vi "Cannon Set.vi"(1 "Cannon Global Data In":T1) -> (0 "Cannon Global Data Out":T1)   [LabVIEW 2012]
uses:
  <vilib>/Rock Robotics/WPI/DriverStation/WPI_DriverStationRobotMode2.ctl
  Extras/Global Data.vi
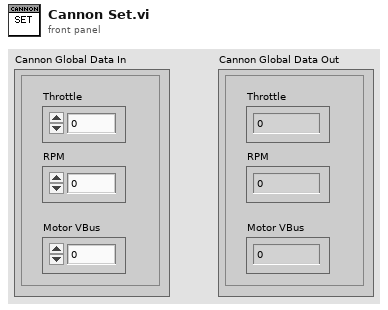
[diagram p1: front panel]
types:
  T1 = cluster{"Throttle":dbl, "RPM":dbl, "Motor VBus":dbl}
  T2 = typedef "WPI_DriverStationRobotMode2.ctl" = enum16{"Autonomous Disabled", "Autonomous Enabled", "Teleop Disabled", "Teleop Enabled", "Timeout", "Finish", "Test Disabled", "Test Enabled"}
  T3 = typedef "WPI_MotorControlDeviceRef.ctl" = cluster{"DeviceStatus":errorcluster, "Type":enum16{"PWM", "CAN"}, "PWM":cluster{"Digital Module":T4, "PWM Channel":T5, "DeadBand":T6}, "CAN":cluster{"Device Number":u8, "Control Mode":T7, "Semaphore":T8, "Max Vout":dbl}, "Invert":bool, "TransformRef":T9, "InvTransformRef":T9}
  T4 = typedef "FPGA_TypedefDigitalModule.ctl" = enum16{"Digital Module 1", "Digital Module 2"}
  T5 = typedef "FPGA_DIOPWMChannel.ctl" = enum8{"PWM 1", "PWM 2", "PWM 3", "PWM 4", "PWM 5", "PWM 6", "PWM 7", "PWM 8", "PWM 9", "PWM 10", "Invalid"}
  T6 = typedef "WPI_PWMDeadband.ctl" = cluster{"Name":string, "maxPositivePwm":i32, "minPositivePwm":i32, "centerPwm":i32, "maxNegativePwm":i32, "minNegativePwm":i32, "angularRange":u16}
  T7 = typedef "WPI_CANJaguar_ControlMode.ctl" = enum8{"Percent VBus", "Current", "Speed", "Position", "Voltage"}
  T8 = typedef "Semaphore RefNum" = refnum<k1>
  T9 = typedef "WPI_PWMTransform_ConPane.ctl" = refnum<vi>
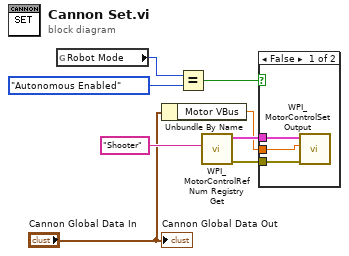
[diagram p0: block diagram]
diagram:
  n1 = global read "Global Data.vi" "Robot Mode"() -> (w4:T2)
  n2 = Unbundle By Name("Cannon Global Data In") -> ("Motor VBus"=w2:dbl)
  n3 = Equal?(x=w4, y=WPI_DriverStationRobotMode2."Autonomous Enabled" ("Robot Mode")) -> (x = y?=w6:bool)
  n4 = call <vilib>:"WPI_MotorControlRefNum Registry Get.vi"("refnum name"="Shooter") -> ("error out"=w1:errorcluster, "MotorControlDevRef"=w3:T3)  [unwired: 9 in]
  n5 = case shown="False" w6 {
    tunnel: w3 -> [w11 _]
    tunnel: w2 -> [w10 _]
    tunnel: w1 -> [w9 _]
    frame False {
      n6 = call <vilib>:"WPI_MotorControlSetOutput.vi"("error in (no error)"=w9, "Output"=w10, "MotorControlDevRef"=w11) -> ()  [unwired: 6 in, 3 out]
    }
    frame True {
    }
  }
  "Cannon Global Data Out" <- "Cannon Global Data In"
